vi "Parse Array.vi"(8 "error in (no error)":errorcluster, 10 "Index In":i32, 11 "JSON String":string) -> (0 "error out":errorcluster, 2 "Index Out":i32, 3 "JSON out":refnum<class "JSON Helper.lvclass">)   [LabVIEW 2016, in "JSON Helper.lvclass"]
uses:
  JSON Helper.lvclass
  Errors/Errors.ctl
  JSON Array/New JSON Array (JSON Data).vi
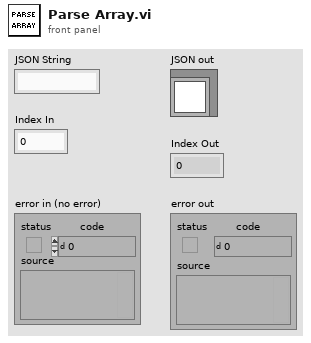
[diagram p1: front panel]
types:
  T1 = typedef "JSON Helper.lvclass/Errors.ctl" = enum16{"No key", "Key path type", "Array OOB", "Type Mismatch", "Invalid Token"}
  T2 = typedef "JSON Helper.lvclass/Token Type.ctl" = enum16{"NONE", "CURLY_OPEN", "CURLY_CLOSE", "SQUARED_OPEN", "SQUARED_CLOSE", "COLON", "COMMA", "STRING", "NUMBER", "TRUE", "FALSE", "NULL"}
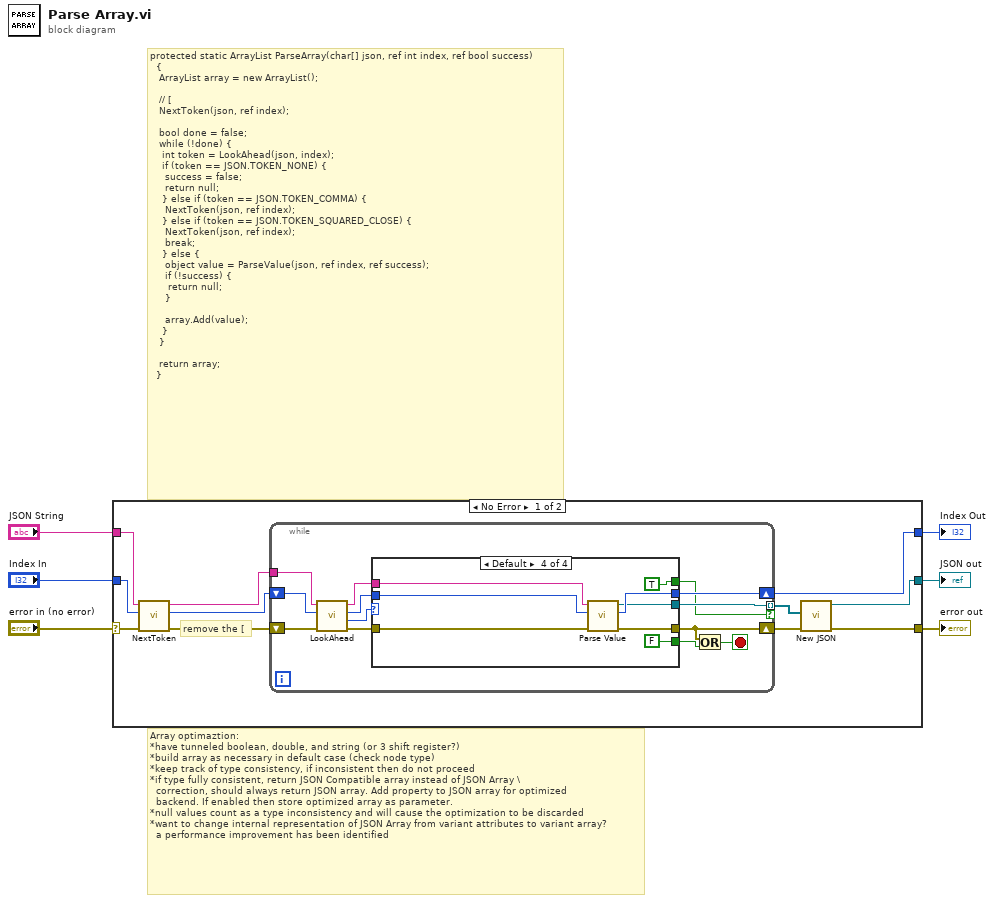
[diagram p0: block diagram]
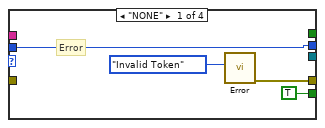
[diagram p2: hidden frame]
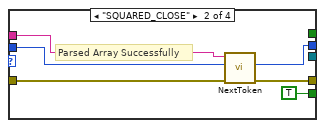
[diagram p3: hidden frame]
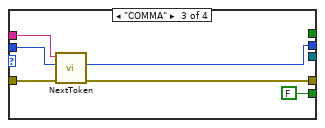
[diagram p4: hidden frame]
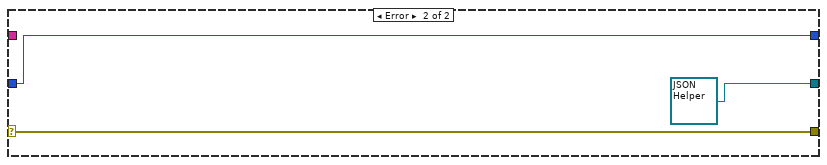
[diagram p5: hidden frame]
diagram:
  # "Array optimaztion:\n*have tunneled boolean, double, and string (or 3 shift register?)\n*build array as necessary in default case (check node type)\n*keep track of type consistency, if inconsistent then do not proceed\n*if type fully consistent, return JSON Compatible array instead of JSON Array \\\n  correction, should always return JSON array. Add property to JSON array for optimized\n  backend. If enabled then store optimized array as parameter.\n*null values count as a type inconsistency and will cause the optimization to be discarded\n*want to change internal representation of JSON Array from variant attributes to variant array?\n  a performance improvement has been identified"
  # "protected static ArrayList ParseArray(char[] json, ref int index, ref bool success)\n\t\t{\n\t\t\tArrayList array = new ArrayList();\n\n\t\t\t// [\n\t\t\tNextToken(json, ref index);\n\n\t\t\tbool done = false;\n\t\t\twhile (!done) {\n\t\t\t\tint token = LookAhead(json, index);\n\t\t\t\tif (token == JSON.TOKEN_NONE) {\n\t\t\t\t\tsuccess = false;\n\t\t\t\t\treturn null;\n\t\t\t\t} else if (token == JSON.TOKEN_COMMA) {\n\t\t\t\t\tNextToken(json, ref index);\n\t\t\t\t} else if (token == JSON.TOKEN_SQUARED_CLOSE) {\n\t\t\t\t\tNextToken(json, ref index);\n\t\t\t\t\tbreak;\n\t\t\t\t} else {\n\t\t\t\t\tobject value = ParseValue(json, ref index, ref success);\n\t\t\t\t\tif (!success) {\n\t\t\t\t\t\treturn null;\n\t\t\t\t\t}\n\n\t\t\t\t\tarray.Add(value);\n\t\t\t\t}\n\t\t\t}\n\n\t\t\treturn array;\n\t\t}"
  n1 = case shown="No Error" "error in (no error)" {
    selector: "error in (no error)" -> [w17 w56]
    tunnel: [w7 w56] -> w5
    tunnel: "Index In" -> [w16 w57]
    tunnel: [w12 w57] -> w3
    tunnel: [w10 refnum<class "JSON Helper.lvclass"> refnum ("JSON out")] -> w1
    tunnel: "JSON String" -> [w11 _]
    frame No Error {
      # "remove the ["
      n2 = call "NextToken.vi"("error in (no error)"=w17, "Index In"=w16, "JSON String"=w11) -> ("error out"=w13:errorcluster, "Index Out"=w15:i32, "JSON String Passthrough"=w14:string)  [unwired: 5 in, 1 out]
      n3 = while {
        shift-right: [w23] -> w12
        shift-left: w15 -> [w29]
        tunnel: w14 -> [w28]
        shift-right: [w20] -> w8
        shift-left: w13 -> [w30]
        tunnel: [w19] -> w9 mode=indexing if=w18
        stop <- w21 stop-if-true
        n4 = call "LookAhead.vi"("error in (no error)"=w30, "Index"=w29, "JSON String"=w28) -> ("error out"=w26:errorcluster, "TOKEN"=w27:T2, "Index Passthrough"=w25:i32, "JSON String Passthrough"=w24:string)  [unwired: 5 in]
        n5 = case shown="Default" w27 {
          tunnel: w26 -> [_ w40 w44 w54]
          tunnel: [TRUE TRUE FALSE FALSE] -> w22
          tunnel: w25 -> [w33 w39 w45 w53]
          tunnel: w24 -> [_ w38 w46 w52]
          tunnel: [w33 w36 w42 w51] -> w23
          tunnel: [w32 w37 w43 w49] -> w20
          tunnel: [_ _ _ w48] -> w19
          tunnel: [_ _ _ TRUE] -> w18
          frame "NONE" {
            # "Error"
            n6 = call "Error.vi"(9:Errors."Invalid Token") -> ("error out"=w32:errorcluster)  [unwired: 9 in]
          }
          frame "SQUARED_CLOSE" {
            # "Parsed Array Successfully"
            n7 = call "NextToken.vi"("error in (no error)"=w40, "Index In"=w39, "JSON String"=w38) -> ("error out"=w37:errorcluster, "Index Out"=w36:i32)  [unwired: 5 in, 2 out]
          }
          frame "COMMA" {
            n8 = call "NextToken.vi"("error in (no error)"=w44, "Index In"=w45, "JSON String"=w46) -> ("error out"=w43:errorcluster, "Index Out"=w42:i32)  [unwired: 5 in, 2 out]
          }
          frame Default {
            n9 = call "Parse Value.vi"("error in (no error)"=w54, "Index In"=w53, "JSON String"=w52) -> ("error out"=w49:errorcluster, "Index Out"=w51:i32, "JSON out"=w48:refnum<class "JSON Helper.lvclass">)  [unwired: 6 in]
          }
        }
        n10 = Or(x=w20, y=w22) -> (x .or. y?=w21:bool)
      }
      n11 = call-poly "New JSON.vi"("error in (no error)"=w8, "JSON Datatypes"=w9) -> ("error out"=w7:errorcluster, "JSON Array out"=w10:refnum<class "JSON Helper.lvclass">)  [unwired: 8 in]
    }
    frame Error {
    }
  }
  "error out" <- w5
  "Index Out" <- w3
  "JSON out" <- w1
